vi "fpga_Locate Memory.vi"(0 "pick-up signal? (F)":bool, 1 "number of channels":T1 items=["1"=1, "2"=2, "3"=3, "4"=4, "5"=5, "6"=6, "7"=7, "8"=8, "9"=9, "10"=10, "11"=11, "12"=12, "13"=13, "14"=14, "15"=15, "16"=16], 2 "memory info of curve":T2, 5 "G":fxp<+/-,48,24>, 7 "Gs":fxp<+/-,48,24>, 9 "input valid? (T)":bool) -> (3 "integrate?":bool, 4 "dt/T":fxp<+/-,32,1>, 6 "channel index":u8, 8 "pick-up signal?":bool, 10 "output valid":bool, 14 "ready for input":bool, 15 "error":i32)   [LabVIEW 2012, in "NI_EP_Protection_FPGA.lvlib"]
uses:
  <vilib>/addons/Electrical Power/Protection/NI_EP_Protection_FPGA.lvlib
  <vilib>/addons/Electrical Power/Protection/Inverse Time Delay/subVIs/ep_Curve Memory.ctl
  <vilib>/addons/Electrical Power/PQ/Resampling/FPGA/subVIs/fpga_NofCH.ctl
  <vilib>/rvi/FXPMathLib/FxpDiv/subVIs/nifxpmath_Div_SimConfig.ctl
  <vilib>/rvi/FXPMathLib/FxpDiv/simVIs/DllFxpDivTemp_sub.vi
  <vilib>/rvi/DataTransferAndStorage/Container/Common/niFpgaContainerExecOnDevCompGetState.vi
  <vilib>/rvi/DataTransferAndStorage/Container/Common/niFpgaContainerGetUniqueNameForEmu.vi
  <vilib>/rvi/Memory/Memory_Emulation/niFpgaMemoryEmulationCacheClearOnFirstRun.vi
  <vilib>/rvi/Memory/Memory_Emulation/nirvimemoryEmulationManagerCache_MakeExclusive.vi
  <vilib>/rvi/Memory/Memory_Emulation/niFpgaMemoryEmulationValidateCache.vi
  <vilib>/rvi/Memory/Memory_Emulation/nirvimemoryEmulationManagerCache_ReleaseExclusive.vi
  <vilib>/rvi/Memory/Memory_Emulation/nirvimemoryEmulationManagerCache_InsertValue.vi
  <vilib>/Utility/error.llb/Clear Errors.vi
  <vilib>/rvi/Memory/Memory_Emulation/nirvimemoryEmulationManagerCache_GetValue.vi
  <vilib>/rvi/FXPMathLib/FxpDiv/XNode/nifxpmath_Div.xnode
  <vilib>/rvi/FXPMathLib/FxpSub/XNode/nifxpmath_Sub.xnode
  <vilib>/rvi/FXPMathLib/FxpMul/XNode/nifxpmath_Multiplier.xnode
  <vilib>/rvi/FXPMathLib/FxpAdd/XNode/nifxpmath_Add.xnode
  <vilib>/rvi/DataTransferAndStorage/Container/XNode/niFpgaContainer.xnode
  <vilib>/rvi/Memory/Memory_Emulation/niFpgaMemoryEmulationRefIn.vi
  <vilib>/rvi/FXPMathLib/basic elements/FxpDiscreteDelay/XNode/nifxpmath_DiscreteDelay.xnode
  <vilib>/rvi/FXPMathLib/sim/FxpSim.dll
  <vilib>/addons/Electrical Power/Protection/NI_EP_Protection.lvlib
  <vilib>/addons/Electrical Power/PQ/Resampling/NI_EP_Resample_FPGA.lvlib
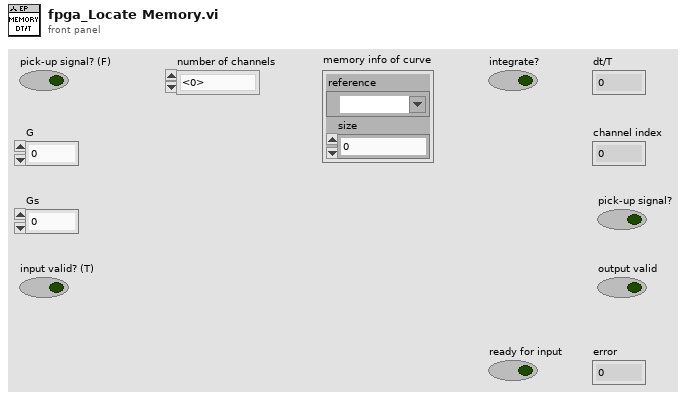
[diagram p1: front panel]
types:
  T1 = typedef "NI_EP_Resample_FPGA.lvlib/fpga_NofCH.ctl" = u8
  T2 = typedef "NI_EP_Protection.lvlib/ep_Curve Memory.ctl" = cluster{"reference":refnum<k21>, "size":u16}
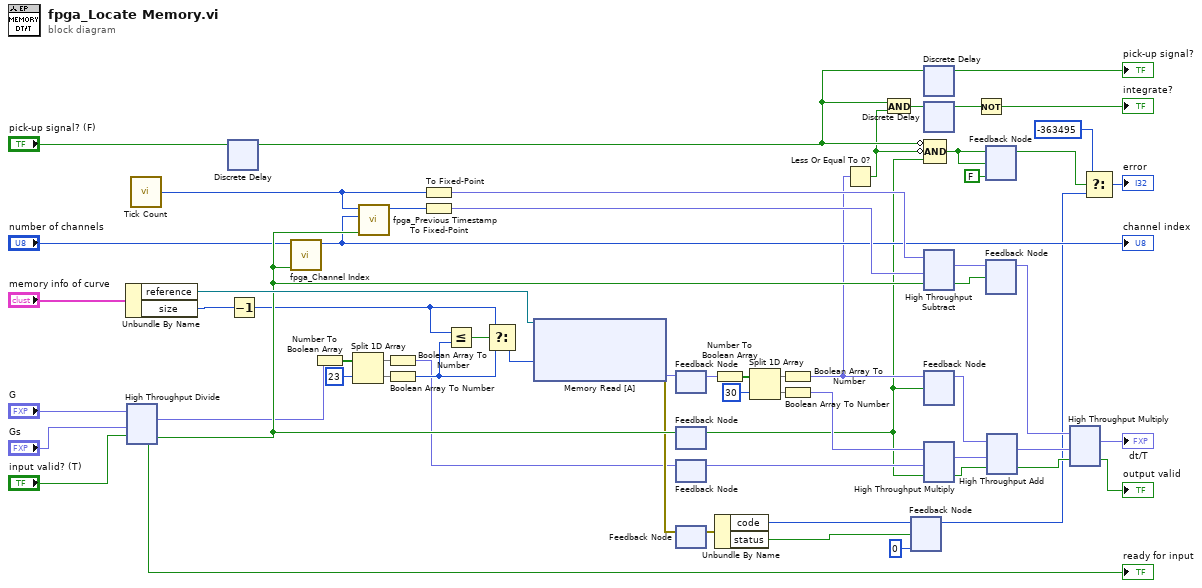
[diagram p0: block diagram]
diagram:
  n1 = Unbundle By Name("memory info of curve") -> ("reference"=w48:refnum<k21>, "size"=w49:u16)
  n2 = xnode "High Throughput Divide"("x"="G", "y"="Gs", "input valid"="input valid? (T)") -> ("x/y"=w33:fxp<+/-,32,6>, "output valid"=w42:bool, "ready for input"=→"ready for input":bool)  [unwired: 1 in]
  n3 = call "Tick Count"() -> ("Tick Count(uSec)"=w53:u32)
  n4 = xnode ("Discrete Delay")("D"="pick-up signal? (F)") -> ("Q"=w9:bool)
  n5 = Decrement(x=w49) -> (x-1=w28:u16)
  n6 = call <vilib>:"fpga_Channel Index.vi"("input valid? (T)"=w42, "number of channels"="number of channels") -> ("channel index"=w40:u8)  [unwired: 9 in]
  "channel index" <- w40
  n7 = Number To Boolean Array(number=w33) -> (Boolean array=w21:bool[])
  n8 = Split 1D Array(array=w21, index=23) -> (first subarray=w23:bool[], second subarray=w22:bool[])
  n9 = call <vilib>:"fpga_Previous Timestamp.vi"("input valid? (T)"=w42, "channel index"=w40, "timestamp"=w53) -> ("previous timestamp"=w41:u32)  [unwired: 8 in]
  n10 = Boolean Array To Number(Boolean array=w23) -> (number=w24:fxp<+,23,0>)
  n11 = Boolean Array To Number(Boolean array=w22) -> (number=w27:u16)
  n12 = To Fixed-Point(number=w53) -> (fixed-point=w45:fxp<+,32,32>)  [unwired: 1 in]
  n13 = To Fixed-Point(number=w41) -> (fixed-point=w43:fxp<+,32,32>)  [unwired: 1 in]
  n14 = Less Or Equal?(x=w28, y=w27) -> (x <= y?=w26:bool)
  n15 = Select(t=w28, s=w26, f=w27) -> (s? t:f=w39:u16)
  n16 = xnode ("Memory Read [A]")("Address"=w39, "Memory In"=w48) -> ("Data"=w11:fxp<+,51,51>, "error out"=w37:errorcluster)  [unwired: 1 in, 1 out]
  n17 = feedback #1() -> (w14:fxp<+,51,51>)  [unwired: 1 in]
  n18 = feedback-in #1(w11) -> ()
  n19 = feedback #2() -> (w7:bool)  [unwired: 1 in]
  n20 = feedback-in #2(w42) -> ()
  n21 = feedback #3() -> (w12:fxp<+,23,0>)  [unwired: 1 in]
  n22 = feedback-in #3(w24) -> ()
  n23 = feedback #4() -> (w38:errorcluster)  [unwired: 1 in]
  n24 = feedback-in #4(w37) -> ()
  n25 = Number To Boolean Array(number=w14) -> (Boolean array=w15:bool[])
  n26 = Unbundle By Name(w38) -> ("code"=w61:i32, "status"=w60:bool)
  n27 = Split 1D Array(array=w15, index=30) -> (first subarray=w17:bool[], second subarray=w18:bool[])
  n28 = Boolean Array To Number(Boolean array=w17) -> (number=w10:fxp<+/-,30,-10>)
  n29 = Boolean Array To Number(Boolean array=w18) -> (number=w19:fxp<+/-,21,-17>)
  n30 = Less Or Equal To 0?(x=w10) -> (x <= 0?=w1:bool)
  n31 = And(x=w9, y=w1) -> (x .and. y?=w50:bool)
  n32 = feedback #5(0 ("code")) -> (w8:i32)
  n33 = feedback-in #5(w61, w60) -> ()
  n34 = xnode ("Discrete Delay")("D"=w9) -> ("Q"=→"pick-up signal?":bool)
  n35 = xnode ("Discrete Delay")("D"=w50) -> ("Q"=w51:bool)
  n36 = Compound Arithmetic op=AND(invert w9, invert w1, w7) -> (w5:bool)
  n37 = xnode ("High Throughput Subtract")("x"=w45, "y"=w43, "input valid"=w42) -> ("x-y"=w46:fxp<+,18,18>, "output valid"=w44:bool)  [unwired: 1 in, 1 out]
  n38 = feedback #6() -> (w25:fxp<+/-,30,-10>)  [unwired: 1 in]
  n39 = feedback-in #6(w10, w7) -> ()
  n40 = xnode ("High Throughput Multiply")("x"=w19, "y"=w12, "input valid"=w7) -> ("x*y"=w30:fxp<+/-,26,-17>, "output valid"=w29:bool)  [unwired: 1 in, 1 out]
  n41 = Not(x=w51) -> (.not. x?=→"integrate?":bool)
  n42 = feedback #7(FALSE) -> (w3:bool)
  n43 = feedback-in #7(w5, w5) -> ()
  n44 = feedback #8() -> (w13:fxp<+,18,18>)  [unwired: 1 in]
  n45 = feedback-in #8(w46, w44) -> ()
  n46 = xnode ("High Throughput Add")("x"=w25, "y"=w30, "input valid"=w29) -> ("x+y"=w32:fxp<+/-,33,-10>, "output valid"=w31:bool)  [unwired: 1 in, 1 out]
  n47 = xnode ("High Throughput Multiply")("x"=w13, "y"=w32, "input valid"=w31) -> ("x*y"=→"dt/T":fxp<+/-,32,1>, "output valid"=→"output valid":bool)  [unwired: 1 in, 1 out]
  n48 = Select(t=-363495 ("code"), s=w3, f=w8) -> (s? t:f=→"error":i32)
